vi "create cycleresult table.vi"() -> ()   [LabVIEW 2016]
uses:
  <vilib>/addons/database/Connection.llb/DB Tools Open Connec (String).vi
  <vilib>/addons/database/Connection.llb/Conn Execute.vi
  <vilib>/addons/database/Recordset.llb/Rec Destroy - Connection.vi
  <vilib>/addons/database/NI_Database_API.lvlib
panel:
  out "error out":errorcluster
  out "error out 2":errorcluster
  out "error out 5":errorcluster
  in  "error in (no error)":errorcluster
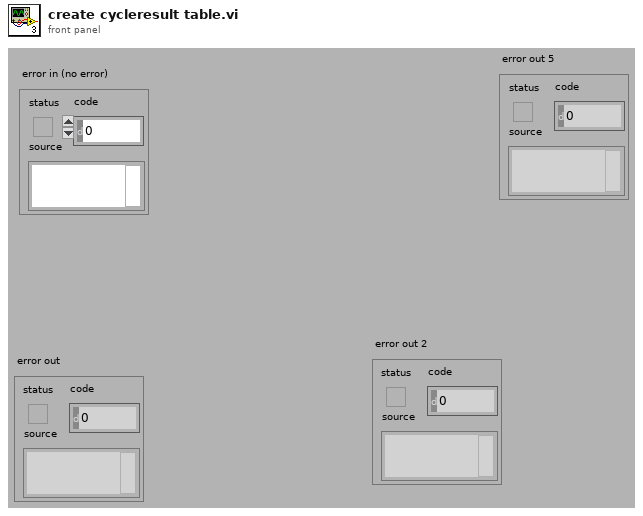
[diagram p1: front panel]
types:
  T1 = typedef "NI_Database_API.lvlib/Conn ObjectReference.ctl" = refnum<k1>
  T2 = typedef "NI_Database_API.lvlib/Rec ObjectReference.ctl" = refnum<k1>
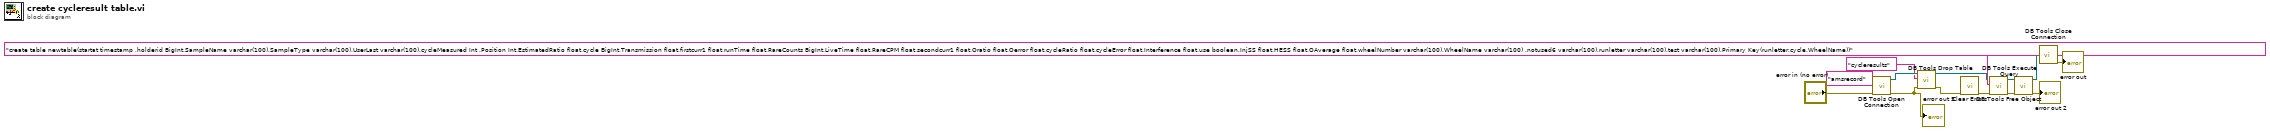
[diagram p0: block diagram]
diagram:
  n1 = call-poly <vilib>:"DB Tools Open Connection.vi"("error in (no error)"="error in (no error)", "connection information"="amsrecord") -> ("error out"=w5:errorcluster, "connection reference"=w3:T1)  [unwired: 6 in]
  "error out 5" <- w5
  n2 = call <vilib>:"DB Tools Drop Table.vi"("error in (no error)"=w5, "table"="cycleresults", "connection reference"=w3) -> ("error out"=w4:errorcluster, "connection reference out"=w2:T1)  [unwired: 5 in]
  n3 = call <vilib>:"Clear Errors.vi"("error in (no error)"=w4) -> ("error out"=w8:errorcluster)  [unwired: 5 in, 1 out]
  n4 = call-poly <vilib>:"DB Tools Execute Query.vi"("error in (no error)"=w8, "SQL query"="create table newtable(startat timestamp ,holderid BigInt,SampleName varchar(100),SampleType varchar(100),UserLast varchar(100),cycleMeasured Int ,Position Int,EstimatedRatio float,cycle BigInt,Transmission float,firstcurr1 float,runTime float,RareCounts BigInt,LiveTime float,RareCPM float,secondcurr1 float,Oratio float,Oerror float,cycleRatio float,cycleError float,Interference float,use boolean,InjSS float,HESS float,OAverage float,wheelNumber varchar(100),WheelName varchar(100) ,notused6 varchar(100),runletter varchar(100),test varchar(100),Primary Key(runletter,cycle,WheelName))" ("concatenated string"), "connection reference"=w2) -> ("error out"=w11:errorcluster, "recordset reference"=w12:T2)  [unwired: 5 in]
  n5 = call-poly <vilib>:"DB Tools Free Object.vi"("error in (no error)"=w11, "recordset reference"=w12) -> ("error out"=→"error out 2":errorcluster, "connection reference"=w10:T1)  [unwired: 8 in]
  n6 = call <vilib>:"DB Tools Close Connection.vi"("connection reference"=w10) -> ("error out"=→"error out":errorcluster)  [unwired: 6 in]
